vi "Last Log.vi"() -> ()   [LabVIEW 2009]
panel:
  out "temperature":timestamp
  out "cryogen":timestamp
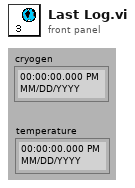
[diagram p1: front panel]
diagram:
